vi "TestVI.vi"() -> ()   [LabVIEW 2011]
panel:
  out "Boolean 4":bool
  out "Boolean 3":bool
  out "Elapsed Time (s)":dbl
  out "Boolean 2":bool
  in  "Boolean":bool
  in  "HMI1 Lock":u8
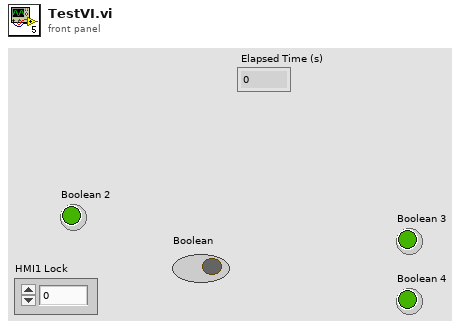
[diagram p1: front panel]
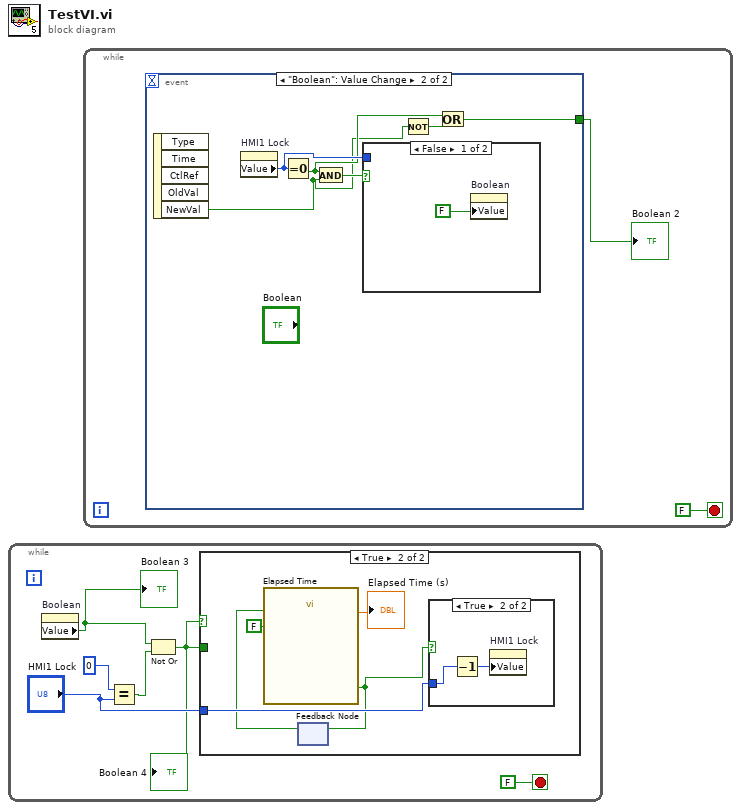
[diagram p0: block diagram]
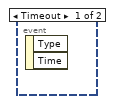
[diagram p4: hidden frame]
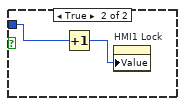
[diagram p5: hidden frame]
diagram:
  n1 = while {
    stop <- FALSE stop-if-true
    n2 = property on="Boolean" class="Bool (strict)"() -> ("Value"=w1:bool)  [unwired: 2 in, 2 out]
    "Boolean 3" <- w1
    n3 = Equal?(x=u8 0, y="HMI1 Lock") -> (x = y?=w3:bool)
    n4 = Not Or(1:w3, 2:w1) -> (0:w2:bool)
    "Boolean 4" <- w2
    n5 = case shown="True" w2 {
      tunnel: "HMI1 Lock" -> [_ w11]
      tunnel: w2 -> [_ _]
      frame False {
      }
      frame True {
        n6 = feedback #1() -> (w7:bool)  [unwired: 1 in]
        n7 = call "Elapsed Time"("Reset"=w7, "Auto Reset"=FALSE) -> ("Elapsed Time (s)"=→"Elapsed Time (s)":dbl, "Time has Elapsed"=w8:bool)  [unwired: 10 in, 6 out]
        n8 = feedback-in #1(w8) -> ()
        n9 = case shown="True" w8 {
          tunnel: w11 -> [_ w12]
          frame False {
          }
          frame True {
            n10 = Decrement(x=w12) -> (x-1=w13:u8)
            n11 = property on="HMI1 Lock" class="DigNum (strict)"("Value"=w13) -> ()  [unwired: 2 in, 2 out]
          }
        }
      }
    }
  }
  n12 = while {
    stop <- FALSE stop-if-true
    n13 = event shown="[1] \"Boolean\": Value Change" {
      selector: _ -> [_ _]
      dyn-events: _ -> [_ _]
      timeout: _ -> [_ _]
      tunnel: [_ w16] -> w14
      event Timeout {
        n14 = event-data() -> ()  [unwired: 1 in, 2 out]
      }
      event "Boolean": Value Change {
        n15 = event-data() -> ("NewVal"=w17:bool)  [unwired: 1 in, 4 out]
        n16 = property on="HMI1 Lock" class="DigNum (strict)"() -> ("Value"=w20:u8)  [unwired: 2 in, 2 out]
        n17 = Equal To 0?(x=w20) -> (x = 0?=w19:bool)
        n18 = And(x=w19, y=w17) -> (x .and. y?=w21:bool)
        n19 = case shown="False" w21 {
          tunnel: w20 -> [_ w24]
          frame False {
            n20 = property on="Boolean" class="Bool (strict)"("Value"=FALSE) -> ()  [unwired: 2 in, 2 out]
          }
          frame True {
            n21 = Increment(x=w24) -> (x+1=w23:u8)
            n22 = property on="HMI1 Lock" class="DigNum (strict)"("Value"=w23) -> ()  [unwired: 2 in, 2 out]
          }
        }
        n23 = Not(x=w17) -> (.not. x?=w18:bool)
        n24 = Or(x=w19, y=w18) -> (x .or. y?=w16:bool)
      }
    }
    "Boolean 2" <- w14
  }
